vi "Autonomous Independent.vi"   [LabVIEW 2019]
doc: "This VI is called when autonomous begins, and will automatically be terminated when autonomous ends. You can carry out timed or sensor driven robot movement independently without needing to return to the caller."
uses:
  <vilib>/Rock Robotics/WPI/ThirdParty/Phoenix-LabVIEW/Motor Controller/Controls/CTRE_Phoenix_MotorControl_ControlMode.ctl
  <vilib>/Rock Robotics/WPI/ThirdParty/Phoenix-LabVIEW/Motor Controller/Controls/CTRE_Phoenix_MotorControl_NeutralMode.ctl
  <vilib>/Rock Robotics/Network Tables/NT Read String.vi
  <vilib>/Rock Robotics/Network Tables/NT Write Number.vi
  <vilib>/Rock Robotics/Network Tables/NT Read Number.vi
  <vilib>/addons/control/pid/pid.llb/PID (DBL).vi
  <vilib>/addons/control/pid/NI_PID_pid.lvlib
types:
  T1 = cluster{"proportional gain (Kc)":dbl, "integral time (Ti, min)":dbl, "derivative time (Td, min)":dbl}
  T2 = typedef "CTRE_Phoenix_MotorControl_NeutralMode.ctl" = enum8{"EEPROMSetting", "Override to Coast", "Override to Brake"}
  T3 = typedef "CTRE_Phoenix_MotorControl_ControlMode.ctl" = u16
  T4 = typedef "WPI_MotorControlDeviceRef.ctl" = cluster{"DeviceStatus":errorcluster, "Type":T5, "PWM":cluster{"PWM Channel":T6, "DeadBand":T7}, "CAN":cluster{"Device Number":u8, "SetOutput VI Ref":variant, "GetOutput VI Ref":variant, "Enable VI Ref":variant, "Disable VI Ref":variant, "Data":variant}, "Invert":bool, "DIO PWM":cluster{"PWM \"Enable\" Channel":T6, "DIOChannel":T8, "PWM Rate":dbl}}
  T5 = typedef "WPI_MotorControlType.ctl" = enum16{"PWM", "CAN", "DIO PWM"}
  T6 = typedef "FPGA_DIOPWMChannel.ctl" = enum8{"PWM 0", "PWM 1", "PWM 2", "PWM 3", "PWM 4", "PWM 5", "PWM 6", "PWM 7", "PWM 8", "PWM 9", "PWM MXP 0", "PWM MXP 1", "PWM MXP 2", "PWM MXP 3", "PWM MXP 4", "PWM MXP 5", "PWM MXP 6", "PWM MXP 7", "PWM MXP 8", "PWM MXP 9", "Invalid"}
  T7 = typedef "WPI_PWMDeadband.ctl" = cluster{"Name":string, "maxPositivePwm":i32, "minPositivePwm":i32, "centerPwm":i32, "maxNegativePwm":i32, "minNegativePwm":i32, "angularRange":u16}
  T8 = typedef "FPGA_DIOChannel.ctl" = enum8{"DIO 0", "DIO 1", "DIO 2", "DIO 3", "DIO 4", "DIO 5", "DIO 6", "DIO 7", "DIO 8", "DIO 9", "DIO MXP 0", "DIO MXP 1", "DIO MXP 2", "DIO MXP 3", "DIO MXP 4", "DIO MXP 5", "DIO MXP 6", "DIO MXP 7", "DIO MXP 8", "DIO MXP 9", "DIO MXP 10", "DIO MXP 11", "DIO MXP 12", "DIO MXP 13", "DIO MXP 14", "DIO MXP 15", "SPI Port CS1", "SPI Port CS2", "SPI Port CS3", "SPI Port MISO", "SPI Port MOSI", "Invalid"}
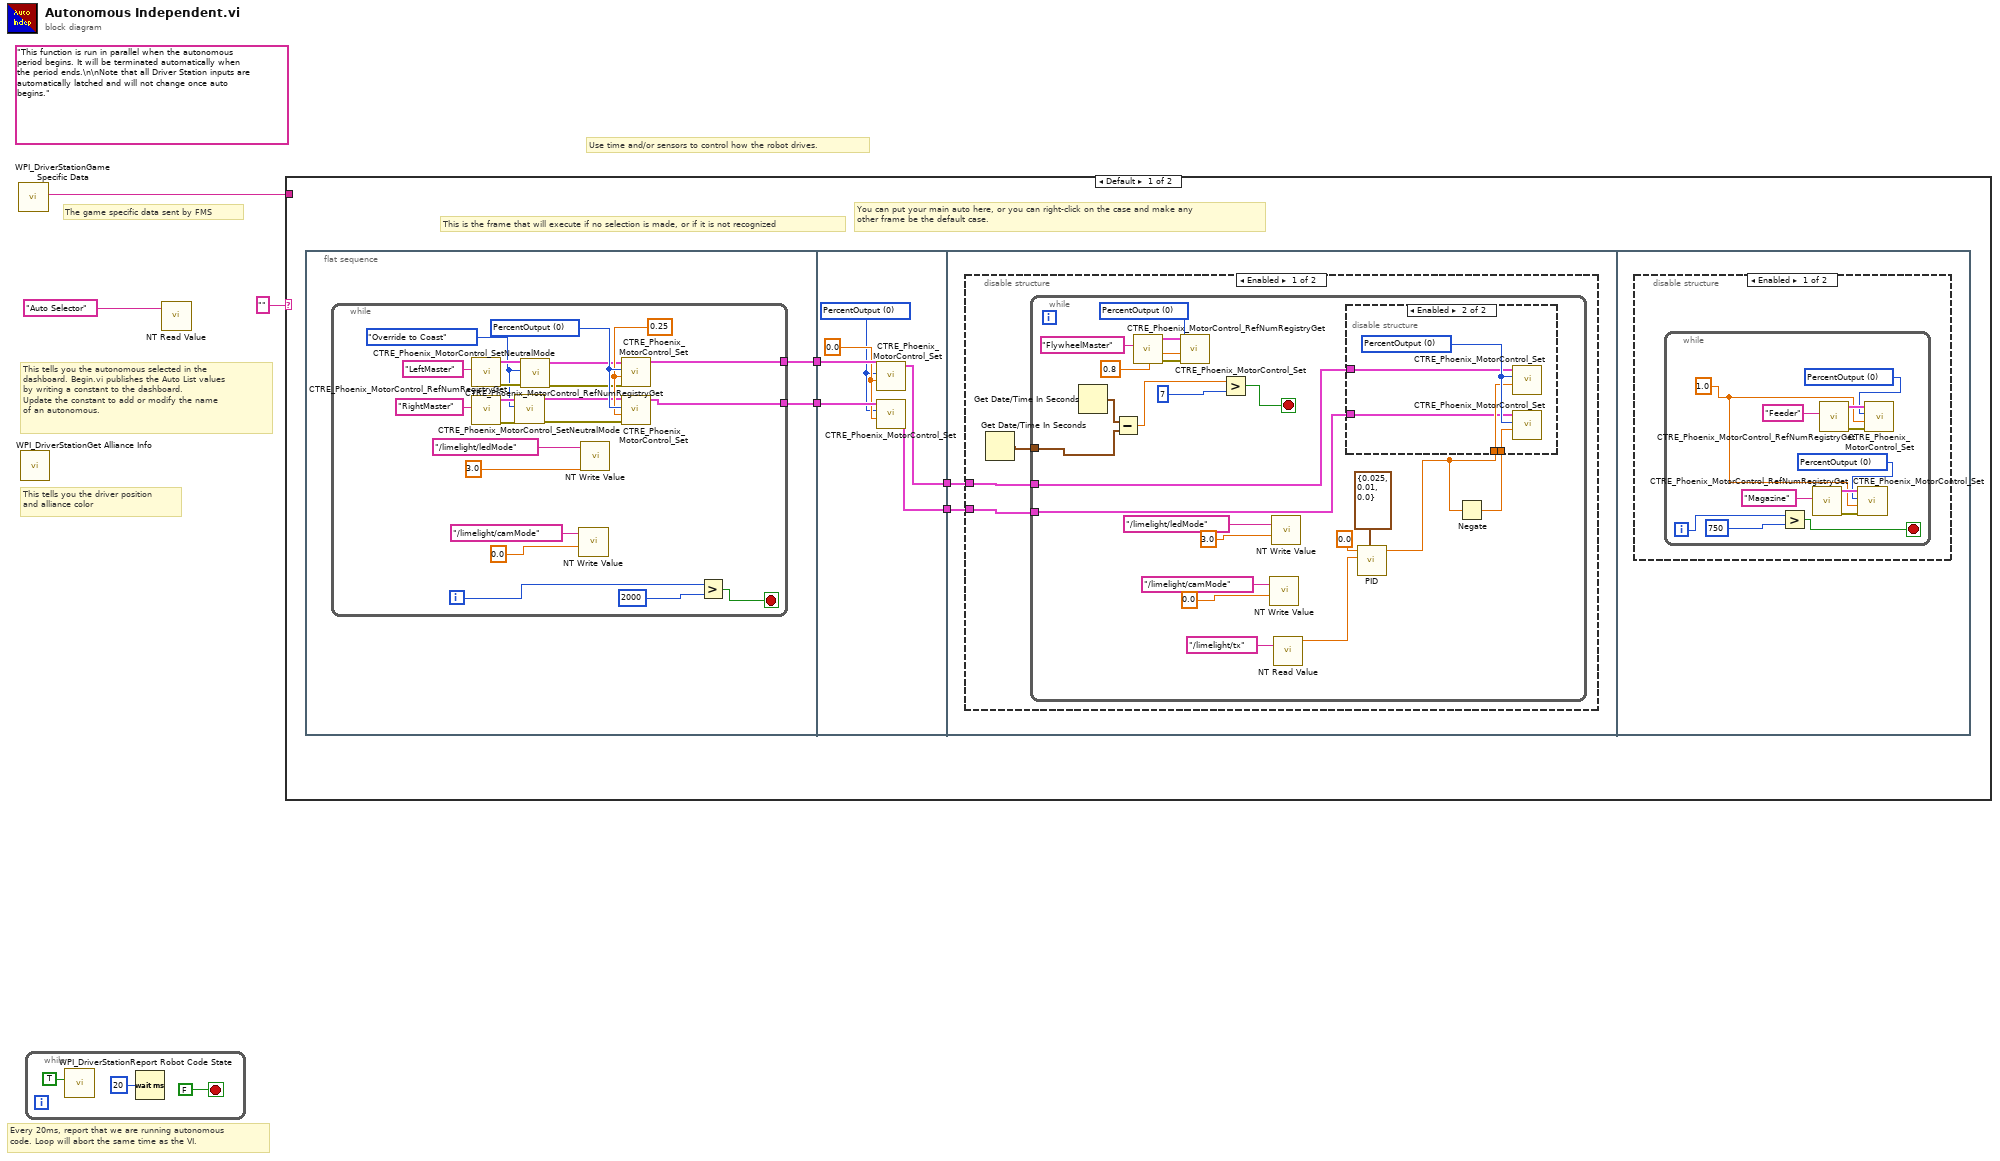
[diagram p0: block diagram]
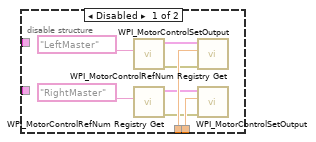
[diagram p2: hidden frame]
diagram:
  (unwired) "This function is run in parallel when the autonomous period begins. It will be terminated automatically when the period ends.\n\nNote that all Driver Station inputs are automatically latched and will not change once auto begins."
  # "The game specific data sent by FMS"
  # "This tells you the autonomous selected in the \ndashboard. Begin.vi publishes the Auto List values\nby writing a constant to the dashboard.\nUpdate the constant to add or modify the name\nof an autonomous."
  # "Every 20ms, report that we are running autonomous\ncode. Loop will abort the same time as the VI."
  # "Use time and/or sensors to control how the robot drives."
  # "This tells you the driver position\nand alliance color"
  n1 = call <vilib>:"WPI_DriverStationGame Specific Data.vi"() -> ("Game Specific Data"=w2:string)  [unwired: 11 in]
  n2 = call <vilib>:"WPI_DriverStationGet Alliance Info.vi"() -> ()  [unwired: 12 out]
  n3 = while {
    stop <- FALSE stop-if-true
    n4 = call <vilib>:"WPI_DriverStationReport Robot Code State.vi"("Autonomous"=TRUE) -> ()  [unwired: 10 in, 1 out]
    n5 = Wait (ms)(milliseconds to wait=u32 20) -> ()  [unwired: 1 out]
  }
  n6 = call-poly <vilib>:"NT Read Value.vi"("Name"="Auto Selector") -> ()  [unwired: 9 in, 2 out]
  n7 = case shown="Default" "" {
    tunnel: w2 -> [_ _]
    frame Default {
      # "You can put your main auto here, or you can right-click on the case and make any\nother frame be the default case."
      # "This is the frame that will execute if no selection is made, or if it is not recognized"
      n8 = flat-sequence {
        tunnel: [w12] -> w10
        tunnel: [w11] -> w9
        tunnel: w10 -> [w40]
        tunnel: w9 -> [w39]
        tunnel: [w36] -> w8
        tunnel: [w35] -> w7
        tunnel: w8 -> [w42]
        tunnel: w7 -> [w41]
        frame #0 {
          n9 = while {
            tunnel: [w28] -> w12
            tunnel: [w27] -> w11
            i -> [w30]
            stop <- w26 stop-if-true
            w17 = CTRE_Phoenix_MotorControl_NeutralMode."Override to Coast" ("Motor Control Neutral Mode")
            w31 = 0.25 ("Output")
            w32 = T3 0 items=["PercentOutput"=0, "Position"=1, "Velocity"=2, "Current"=3, "Follower"=5, "MotionProfile"=6, "MotionMagic"=7, "MotionProfileArc"=10, "Disabled"=15] ("Control Mode")
            n10 = call <vilib>:"CTRE_Phoenix_MotorControl_RefNumRegistryGet.vi"("refnum name"="LeftMaster") -> ("error out"=w25:errorcluster, "PhoenixMotorControlDevRef"=w24:T4)  [unwired: 9 in]
            n11 = call <vilib>:"CTRE_Phoenix_MotorControl_RefNumRegistryGet.vi"("refnum name"="RightMaster") -> ("error out"=w23:errorcluster, "PhoenixMotorControlDevRef"=w22:T4)  [unwired: 9 in]
            n12 = call <vilib>:"CTRE_Phoenix_MotorControl_SetNeutralMode.vi"("error in (no error)"=w23, "Motor Control Neutral Mode"=w17, "PhoenixMotorControlDevRef"=w22) -> ("error out"=w18:errorcluster, "PhoenixMotorControlDevRef"=w19:T4)  [unwired: 7 in]
            n13 = call <vilib>:"CTRE_Phoenix_MotorControl_SetNeutralMode.vi"("error in (no error)"=w25, "Motor Control Neutral Mode"=w17, "PhoenixMotorControlDevRef"=w24) -> ("error out"=w20:errorcluster, "PhoenixMotorControlDevRef"=w21:T4)  [unwired: 7 in]
            n14 = call-poly <vilib>:"NT Write Value.vi"("Numeric"=0.0, "Name"="/limelight/camMode") -> ()  [unwired: 9 in, 1 out]
            n15 = call-poly <vilib>:"NT Write Value.vi"("Numeric"=3.0, "Name"="/limelight/ledMode") -> ()  [unwired: 9 in, 1 out]
            n16 = call <vilib>:"CTRE_Phoenix_MotorControl_Set.vi"("error in (no error)"=w20, "Output"=w31, "Control Mode"=w32, "PhoenixMotorControlDevRef"=w21) -> ("PhoenixMotorControlDevRef"=w28:T4)  [unwired: 6 in, 1 out]
            n17 = call <vilib>:"CTRE_Phoenix_MotorControl_Set.vi"("error in (no error)"=w18, "Output"=w31, "Control Mode"=w32, "PhoenixMotorControlDevRef"=w19) -> ("PhoenixMotorControlDevRef"=w27:T4)  [unwired: 6 in, 1 out]
            n18 = Greater?(x=w30, y=2000) -> (0:w26:bool)
          }
        }
        frame #1 {
          w37 = T3 0 items=["PercentOutput"=0, "Position"=1, "Velocity"=2, "Current"=3, "Follower"=5, "MotionProfile"=6, "MotionMagic"=7, "MotionProfileArc"=10, "Disabled"=15] ("Control Mode")
          w38 = 0.0 ("Output")
          n19 = call <vilib>:"CTRE_Phoenix_MotorControl_Set.vi"("Output"=w38, "Control Mode"=w37, "PhoenixMotorControlDevRef"=w40) -> ("PhoenixMotorControlDevRef"=w36:T4)  [unwired: 7 in, 1 out]
          n20 = call <vilib>:"CTRE_Phoenix_MotorControl_Set.vi"("Output"=w38, "Control Mode"=w37, "PhoenixMotorControlDevRef"=w39) -> ("PhoenixMotorControlDevRef"=w35:T4)  [unwired: 7 in, 1 out]
        }
        frame #2 {
          n21 = disable-structure shown="Enabled" {
            disable-tunnel: w42 -> [w45 _]
            disable-tunnel: w41 -> [w44 _]
            frame Enabled {
              n22 = Get Date/Time In Seconds() -> (seconds since 1Jan1904=w43:timestamp)
              n23 = while {
                tunnel: w45 -> [w50]
                tunnel: w44 -> [w49]
                tunnel: w43 -> [w47]
                stop <- w61 stop-if-true
                w64 = T3 0 items=["PercentOutput"=0, "Position"=1, "Velocity"=2, "Current"=3, "Follower"=5, "MotionProfile"=6, "MotionMagic"=7, "MotionProfileArc"=10, "Disabled"=15] ("Control Mode")
                n24 = Get Date/Time In Seconds() -> (seconds since 1Jan1904=w48:timestamp)
                n25 = Subtract(x=w48, y=w47) -> (x-y=w46:dbl)
                n26 = call <vilib>:"CTRE_Phoenix_MotorControl_RefNumRegistryGet.vi"("refnum name"="FlywheelMaster") -> ("error out"=w65:errorcluster, "PhoenixMotorControlDevRef"=w66:T4)  [unwired: 9 in]
                n27 = call <vilib>:"CTRE_Phoenix_MotorControl_Set.vi"("error in (no error)"=w65, "Output"=0.8, "Control Mode"=w64, "PhoenixMotorControlDevRef"=w66) -> ()  [unwired: 6 in, 2 out]
                n28 = Greater?(x=w46, y=7) -> (0:w61:bool)
                n29 = call-poly <vilib>:"NT Write Value.vi"("Numeric"=0.0, "Name"="/limelight/camMode") -> ()  [unwired: 9 in, 1 out]
                n30 = call-poly <vilib>:"NT Write Value.vi"("Numeric"=3.0, "Name"="/limelight/ledMode") -> ()  [unwired: 9 in, 1 out]
                n31 = call-poly <vilib>:"NT Read Value.vi"("Name"="/limelight/tx") -> ("Numeric"=w58:dbl)  [unwired: 9 in, 1 out]
                n32 = call-poly <vilib>:"PID.vi"("PID gains"=T1 {"proportional gain (Kc)"=0.025, "integral time (Ti, min)"=0.01, "derivative time (Td, min)"=0.0}, "process variable"=w58, "setpoint"=0.0) -> ("output"=w59:dbl)  [unwired: 7 in, 1 out]
                n33 = Negate(x=w59) -> (-x=w60:dbl)
                n34 = disable-structure shown="Enabled" {
                  disable-tunnel: w59 -> [w75 w79]
                  disable-tunnel: w60 -> [w74 w78]
                  disable-tunnel: w50 -> [_ w77]
                  disable-tunnel: w49 -> [_ w76]
                  frame Disabled {
                    n35 = call <vilib>:"WPI_MotorControlRefNum Registry Get.vi"("refnum name"="LeftMaster") -> ("error out"=w71:errorcluster, "MotorControlDevRef"=w70:T4)  [unwired: 9 in]
                    n36 = call <vilib>:"WPI_MotorControlRefNum Registry Get.vi"("refnum name"="RightMaster") -> ("error out"=w69:errorcluster, "MotorControlDevRef"=w68:T4)  [unwired: 9 in]
                    n37 = call <vilib>:"WPI_MotorControlSetOutput.vi"("error in (no error)"=w71, "Output"=w75, "MotorControlDevRef"=w70) -> ()  [unwired: 6 in, 3 out]
                    n38 = call <vilib>:"WPI_MotorControlSetOutput.vi"("error in (no error)"=w69, "Output"=w74, "MotorControlDevRef"=w68) -> ()  [unwired: 6 in, 3 out]
                  }
                  frame Enabled {
                    w80 = T3 0 items=["PercentOutput"=0, "Position"=1, "Velocity"=2, "Current"=3, "Follower"=5, "MotionProfile"=6, "MotionMagic"=7, "MotionProfileArc"=10, "Disabled"=15] ("Control Mode")
                    n39 = call <vilib>:"CTRE_Phoenix_MotorControl_Set.vi"("Output"=w79, "Control Mode"=w80, "PhoenixMotorControlDevRef"=w77) -> ()  [unwired: 7 in, 2 out]
                    n40 = call <vilib>:"CTRE_Phoenix_MotorControl_Set.vi"("Output"=w78, "Control Mode"=w80, "PhoenixMotorControlDevRef"=w76) -> ()  [unwired: 7 in, 2 out]
                  }
                }
              }
            }
            frame Disabled {
            }
          }
        }
        frame #3 {
          n41 = disable-structure shown="Enabled" {
            frame Enabled {
              n42 = while {
                i -> [w82]
                stop <- w81 stop-if-true
                w84 = 1.0 ("Output")
                w85 = T3 0 items=["PercentOutput"=0, "Position"=1, "Velocity"=2, "Current"=3, "Follower"=5, "MotionProfile"=6, "MotionMagic"=7, "MotionProfileArc"=10, "Disabled"=15] ("Control Mode")
                w87 = T3 0 items=["PercentOutput"=0, "Position"=1, "Velocity"=2, "Current"=3, "Follower"=5, "MotionProfile"=6, "MotionMagic"=7, "MotionProfileArc"=10, "Disabled"=15] ("Control Mode")
                n43 = Greater?(x=w82, y=750) -> (0:w81:bool)
                n44 = call <vilib>:"CTRE_Phoenix_MotorControl_RefNumRegistryGet.vi"("refnum name"="Magazine") -> ("error out"=w89:errorcluster, "PhoenixMotorControlDevRef"=w90:T4)  [unwired: 9 in]
                n45 = call <vilib>:"CTRE_Phoenix_MotorControl_RefNumRegistryGet.vi"("refnum name"="Feeder") -> ("error out"=w92:errorcluster, "PhoenixMotorControlDevRef"=w91:T4)  [unwired: 9 in]
                n46 = call <vilib>:"CTRE_Phoenix_MotorControl_Set.vi"("error in (no error)"=w89, "Output"=w84, "Control Mode"=w87, "PhoenixMotorControlDevRef"=w90) -> ()  [unwired: 6 in, 2 out]
                n47 = call <vilib>:"CTRE_Phoenix_MotorControl_Set.vi"("error in (no error)"=w92, "Output"=w84, "Control Mode"=w85, "PhoenixMotorControlDevRef"=w91) -> ()  [unwired: 6 in, 2 out]
              }
            }
            frame Disabled {
            }
          }
        }
      }
    }
    frame "v2" {
    }
  }
